vi "2.vi"() -> ()   [LabVIEW 2015]
panel:
  out "Updated Duplicated Points":i32
  out "Update Missing Points":i32
  in  "Current Missing Points":i32
  in  "Previous Producer Iterations":i32
  in  "Producer Iterations":i32
  in  "Current Duplicated Points":i32
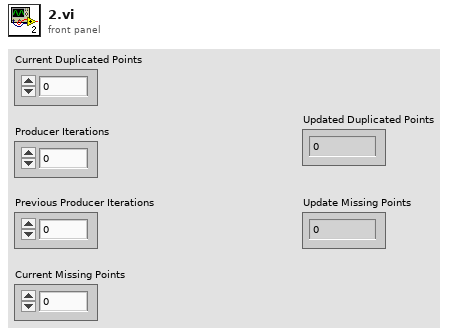
[diagram p1: front panel]
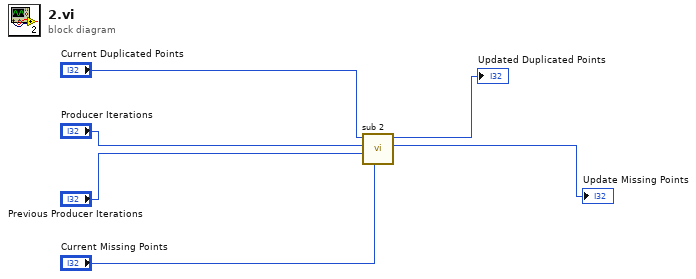
[diagram p0: block diagram]
diagram:
  n1 = call "sub 2.vi"("Current Missing Points"="Current Missing Points", "Previous Producer Iterations"="Previous Producer Iterations", "Producer Iterations"="Producer Iterations", "Current Duplicated Points"="Current Duplicated Points") -> ("Update Missing Points"=→"Update Missing Points":i32, "Updated Duplicated Points"=→"Updated Duplicated Points":i32)  [unwired: 6 in]
